vi "Check if Custom Device is Enabled.vi"(8 "error in":errorcluster, 11 "custom device ref in":T1 format="%.0x") -> (0 "error out":errorcluster, 2 "Custom Device is Enabled":bool, 3 "custom device ref out":T1 format="%.0x")   [LabVIEW 2020, in "AIM ARINC 664 System Explorer.lvlib" / "Implementation.lvlib"]
uses:
  Implementation.lvlib
  <vilib>/NI VeriStand/Custom Device API/Custom Device Item Ref.ctl
  Scripting/AIM ARINC 664 Scripting.lvlib
  <vilib>/NI VeriStand/Custom Device API/Custom Device API.lvlib
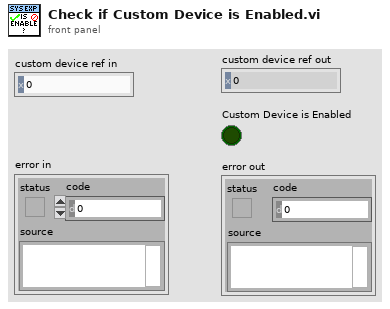
[diagram p1: front panel]
types:
  T1 = typedef "Custom Device API.lvlib/Custom Device Item Ref.ctl" = u64
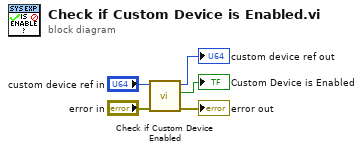
[diagram p0: block diagram]
diagram:
  n1 = call "Check if Custom Device Enabled.vi"("error in"="error in", "custom device ref in"="custom device ref in") -> ("error out"=→"error out":errorcluster, "custom device is enabled"=→"Custom Device is Enabled":bool, "custom device ref out"=→"custom device ref out":T1)  [unwired: 7 in]
